vi "Colour pattern attempt 1.vi"() -> ()   [LabVIEW 2020]
panel:
  out "Yellow":bool
  out "Red":bool
  out "Blue":bool
  out "Green":bool
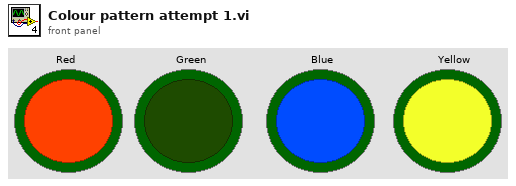
[diagram p1: front panel]
types:
  T1 = enum16{"Left Button", "Center Button", "Right Button", "Window Close"}
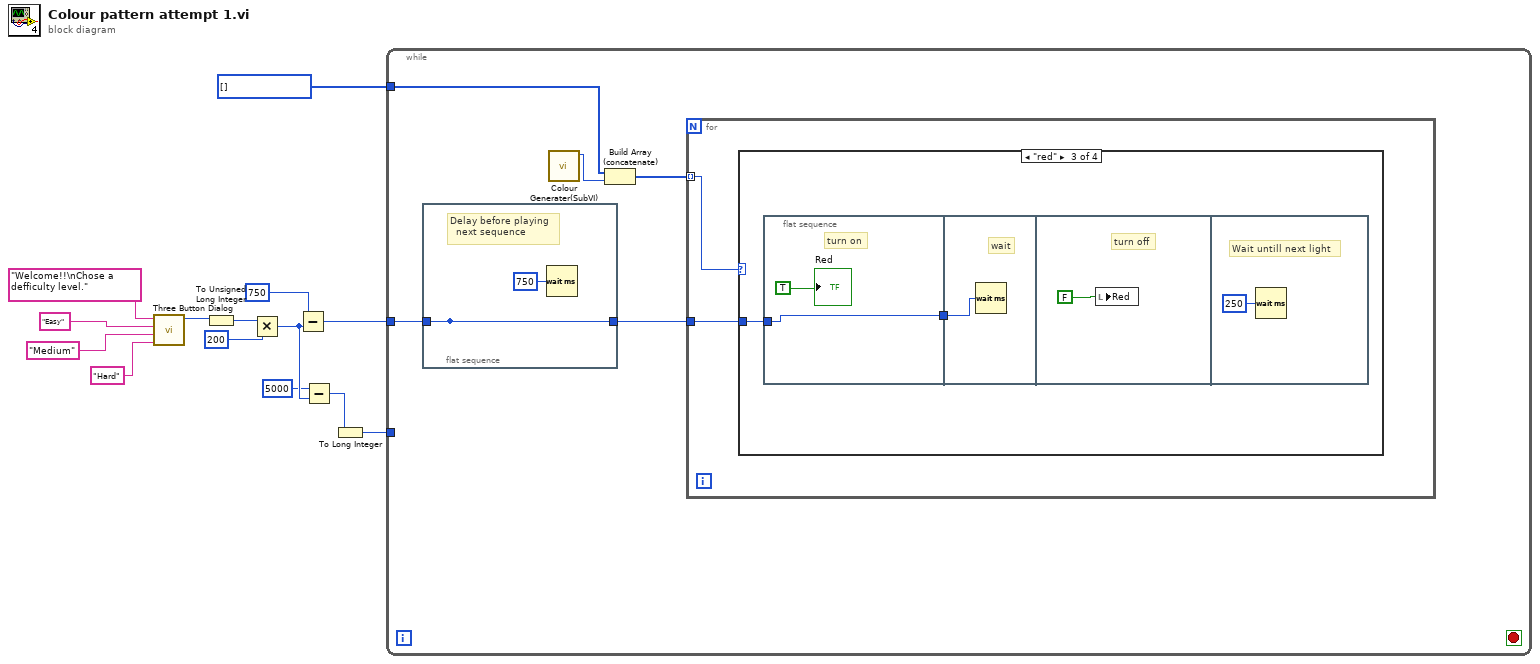
[diagram p0: block diagram]
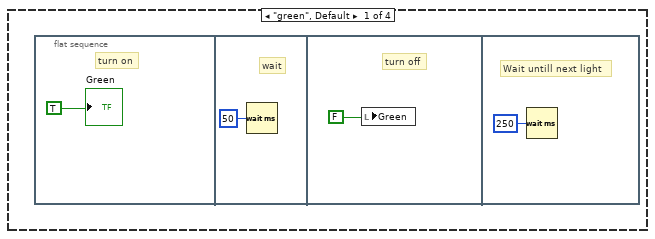
[diagram p2: hidden frame]
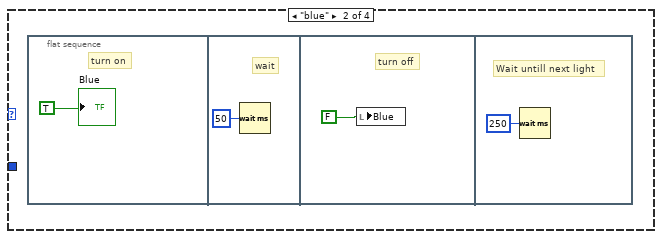
[diagram p3: hidden frame]
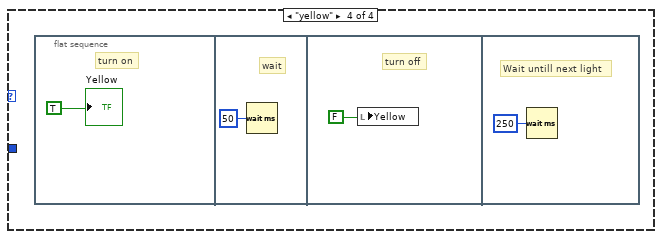
[diagram p4: hidden frame]
diagram:
  w14 = enum16{"green", "blue", "red", "yellow"}[] [] items=["green", "blue", "red", "yellow"]
  n1 = call <vilib>:"Three Button Dialog.vi"("Right Button Text (\"Cancel\")"="Hard" ("Right Button Text (\"Cancel\")"), "Center Button Text (\"No\")"="Medium" ("Center Button Text (\"No\")"), "Left Button Text (\"Yes\")"="Easy" ("Left Button Text (\"Yes\")"), "message"="Welcome!!\nChose a defficulty level.") -> ("Which Button?"=w13:T1)  [unwired: 7 in]
  n2 = To Unsigned Long Integer(number=w13) -> (unsigned 32bit integer=w12:u32)
  n3 = Multiply(x=w12, y=u32 200) -> (x*y=w9:u32)
  n4 = Subtract(x=u32 750, y=w9) -> (x-y=w5:u32)
  n5 = Subtract(x=u32 5000, y=w9) -> (x-y=w7:u32)
  n6 = To Long Integer(number=w7) -> (32bit integer=w6:i32)
  n7 = while {
    tunnel: w14 -> [w17]
    tunnel: w6 -> [_]
    tunnel: w5 -> [w16]
    stop <- _ stop-if-true
    n8 = flat-sequence {
      tunnel: [w20] -> _
      tunnel: w16 -> [w20]
      tunnel: [w20] -> w15
      frame #0 {
        # "Delay before playing\n  next sequence"
        n9 = Wait (ms)(milliseconds to wait=u32 750) -> ()  [unwired: 1 out]
      }
    }
    n10 = call "Colour Generater(SubVI).vi"() -> ("Colour"=w19:enum16{"green", "blue", "red", "yellow"})  [unwired: 11 in]
    n11 = Build Array (concatenate)(w17, w19) -> (w18:enum16{"green", "blue", "red", "yellow"}[])
    n12 = for {
      tunnel: w18 -> [w23] mode=indexing
      tunnel: w15 -> [w22]
      n13 = case shown="\"red\"" w23 {
        tunnel: w22 -> [_ _ w32 _]
        frame "green", Default {
          n14 = flat-sequence {
            frame #0 {
              # "turn on"
              "Green" <- TRUE
            }
            frame #1 {
              # "wait"
              n15 = Wait (ms)(milliseconds to wait=u32 50) -> ()  [unwired: 1 out]
            }
            frame #2 {
              # "turn off"
              n16 = local write "Green"(FALSE) -> ()
            }
            frame #3 {
              # "Wait untill next light"
              n17 = Wait (ms)(milliseconds to wait=u32 250) -> ()  [unwired: 1 out]
            }
          }
        }
        frame "blue" {
          n18 = flat-sequence {
            frame #0 {
              # "turn on"
              "Blue" <- TRUE
            }
            frame #1 {
              # "wait"
              n19 = Wait (ms)(milliseconds to wait=u32 50) -> ()  [unwired: 1 out]
            }
            frame #2 {
              # "turn off"
              n20 = local write "Blue"(FALSE) -> ()
            }
            frame #3 {
              # "Wait untill next light"
              n21 = Wait (ms)(milliseconds to wait=u32 250) -> ()  [unwired: 1 out]
            }
          }
        }
        frame "red" {
          n22 = flat-sequence {
            tunnel: [w34] -> w33
            tunnel: w32 -> [w34]
            tunnel: w33 -> [w36]
            frame #0 {
              # "turn on"
              "Red" <- TRUE
            }
            frame #1 {
              # "wait"
              n23 = Wait (ms)(milliseconds to wait=w36) -> ()  [unwired: 1 out]
            }
            frame #2 {
              # "turn off"
              n24 = local write "Red"(FALSE) -> ()
            }
            frame #3 {
              # "Wait untill next light"
              n25 = Wait (ms)(milliseconds to wait=u32 250) -> ()  [unwired: 1 out]
            }
          }
        }
        frame "yellow" {
          n26 = flat-sequence {
            frame #0 {
              # "turn on"
              "Yellow" <- TRUE
            }
            frame #1 {
              # "wait"
              n27 = Wait (ms)(milliseconds to wait=u32 50) -> ()  [unwired: 1 out]
            }
            frame #2 {
              # "turn off"
              n28 = local write "Yellow"(FALSE) -> ()
            }
            frame #3 {
              # "Wait untill next light"
              n29 = Wait (ms)(milliseconds to wait=u32 250) -> ()  [unwired: 1 out]
            }
          }
        }
      }
    }
  }
